vi "Build core.vi"(6 "Previous Build's Artifacts":refnum<class "Build Artifact.lvclass">[](array[class]), 7 "Progress":refnum<class "Progress.lvclass">, 8 "error in (no error)":errorcluster, 10 "Build Cache":refnum<class "Build Cache.lvclass">, 11 "Build Item in":refnum<class "Run Tests Step.lvclass">) -> (0 "error out":errorcluster, 1 "Explore Path":path, 2 "Build Results":T1, 4 "New Artifacts":refnum<class "Build Artifact.lvclass">[](array[class]))   [LabVIEW 2019, in "Caraya Library.lvlib" / "Run Tests Step.lvclass"]
doc: "Performs all the necessary build actions for the build step.\n\nCopyright: MGI 2016\nAuthor: Derek Trepanier"
uses:
  Run Tests Step.lvclass
  C:/Users/pasca/source/repos/mgi-solution-explorer-extensions/libs/Solution.lvlibp/Solution/Build Item/Build Step.lvclass
  libs/Solution.lvlibp/Solution/Progress/Progress.lvclass
  libs/Solution.lvlibp/Solution/Build Artifact/Build Artifact.lvclass
  libs/Solution.lvlibp/Solution/Build Item/Build Result.ctl
  libs/Solution.lvlibp/Solution/Build Cache/Build Cache.lvclass
  Run Tests Step.lvclass/Run Tests Step.ctl
  libs/Project.lvlibp/Project/Binary File/Binary File.lvclass
  C:/Users/pasca/source/repos/mgi-solution-explorer-extensions/libs/Solution.lvlibp/Solution/Build Artifact/Build Artifact.lvclass
  libs/Solution.lvlibp/Solution/Build Item/Build Step.lvclass
  <vilib>/addons/_JKI Toolkits/Caraya/Caraya.lvlib
  <vilib>/addons/_JKI Toolkits/Caraya/run-tests/Run Test (Scalar Path).vi
  Caraya Library.lvlib
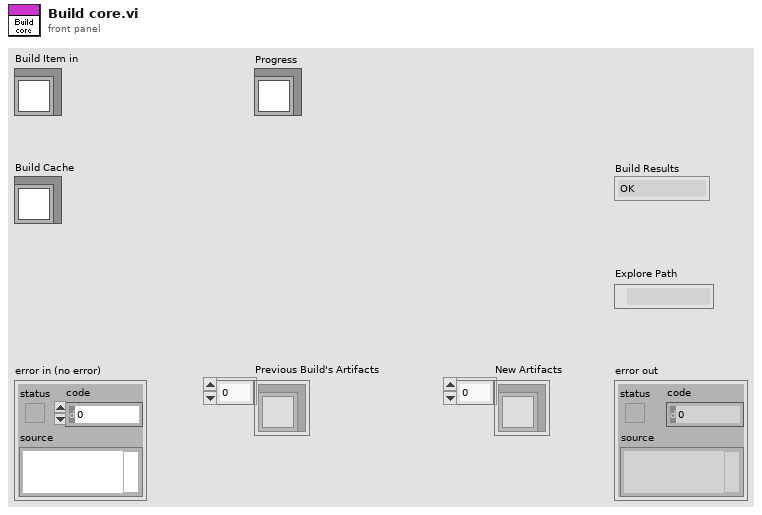
[diagram p1: front panel]
types:
  T1 = typedef "Solution.lvlibp/Build Step.lvclass/Build Result.ctl" = enum16{"OK", "Skipped", "Error"}
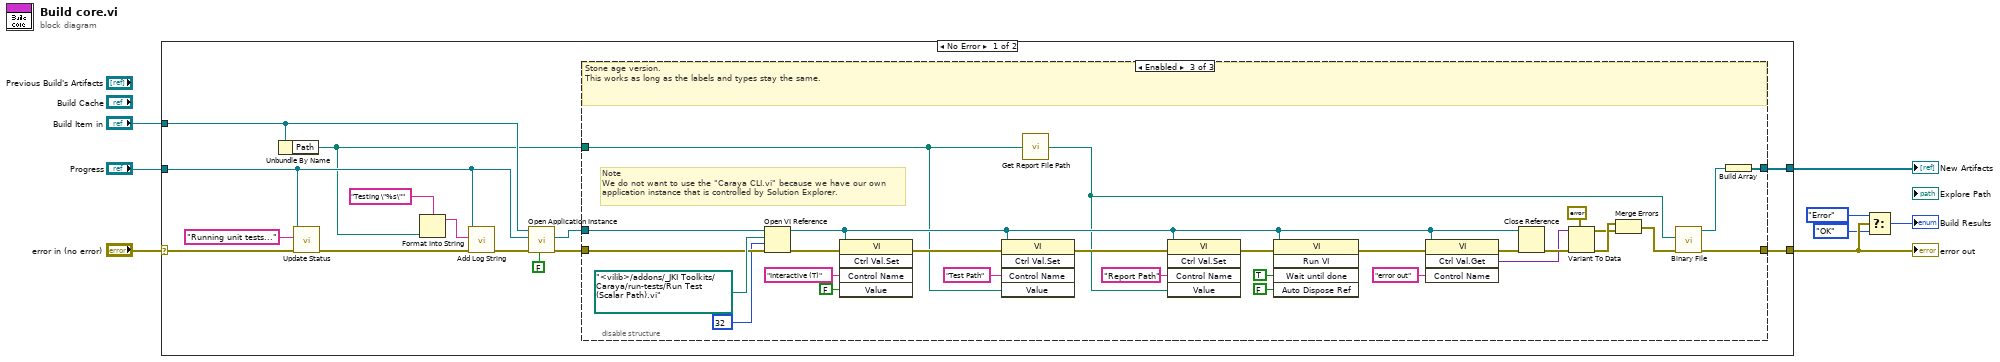
[diagram p0: block diagram]
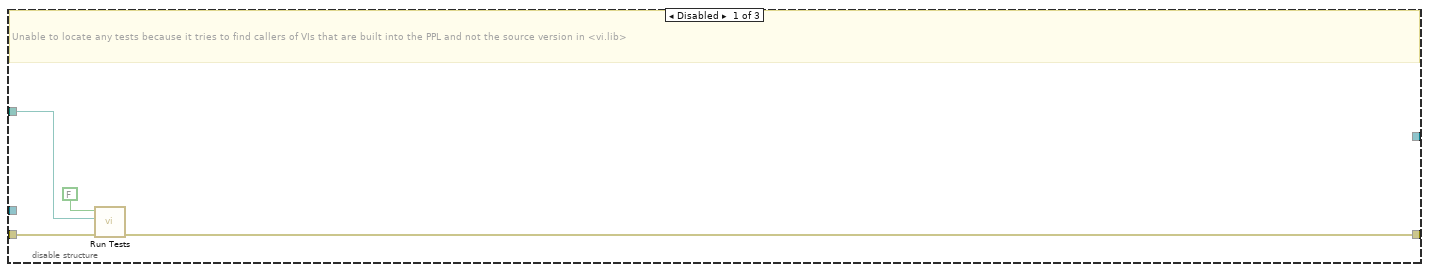
[diagram p2: hidden frame]
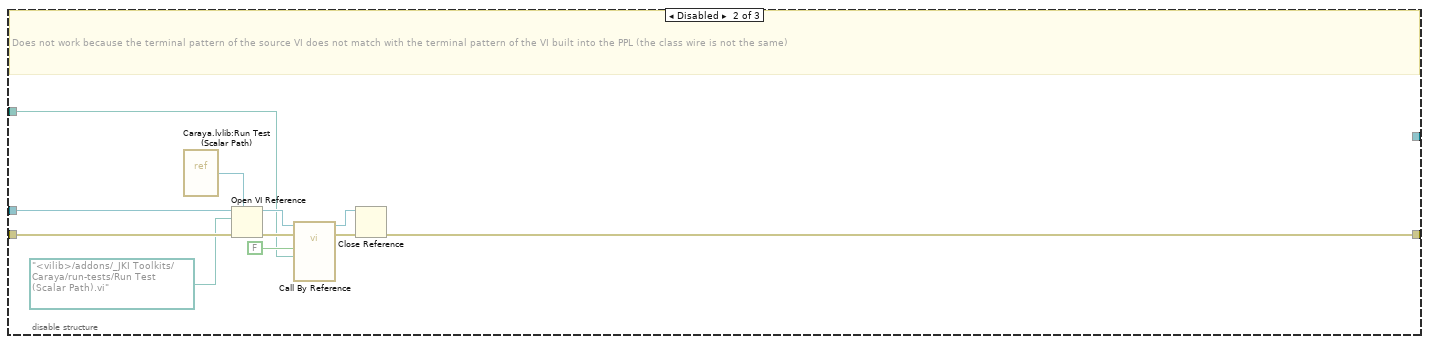
[diagram p3: hidden frame]
diagram:
  n1 = case shown="No Error" "error in (no error)" {
    selector: "error in (no error)" -> [w22 w67]
    tunnel: [w11 w67] -> w5
    tunnel: "Build Item in" -> [w16 _]
    tunnel: "Progress" -> [w15 _]
    tunnel: [w9 _] -> w1
    frame No Error {
      n2 = Unbundle By Name(w16) -> ("Path"=w12:path)
      n3 = call "Update Status.vi"("error in (no error)"=w22, "Status String"="Running unit tests...", "Progress in"=w15) -> ("error out"=w20:errorcluster)  [unwired: 8 in]
      n4 = Format Into String(format string="Testing \"%s\"" ("Log Item"), w12) -> (resulting string=w18:string)  [unwired: 2 in, 1 out]
      n5 = call "Add Log String.vi"("error in (no error)"=w20, "Log Item"=w18, "Progress in"=w15) -> ("error out"=w17:errorcluster)  [unwired: 8 in]
      n6 = call "Open Application Instance.vi"("64 Bit?"=FALSE, "error in (no error)"=w17, "Progress"=w15, "Build Step in"=w16) -> ("error out"=w13:errorcluster, "App ref"=w10:refnum<vi>)  [unwired: 6 in]
      n7 = disable-structure shown="Enabled" {
        disable-tunnel: w13 -> [w26 w37 w65]
        disable-tunnel: w12 -> [w24 w30 w39]
        disable-tunnel: [w23 w29 w51] -> w11
        disable-tunnel: w10 -> [_ w27 w55]
        disable-tunnel: [_ _ w49] -> w9
        frame Disabled {
          # "Unable to locate any tests because it tries to find callers of VIs that are built into the PPL and not the source version in <vi.lib>"
          n8 = call-poly <vilib>:"Run Tests.vi"("error in"=w26, "Test Path"=w24, "Interactive (T)"=FALSE) -> ("error out"=w23:errorcluster)  [unwired: 7 in, 1 out]
        }
        frame Disabled {
          # "Does not work because the terminal pattern of the source VI does not match with the terminal pattern of the VI built into the PPL (the class wire is not the same)"
          n9 = vi-ref "Caraya.lvlib:Run Test (Scalar Path).vi"() -> (w36:refnum<vi>)
          n10 = Open VI Reference(type specifier VI Refnum (for type only)=w36, application reference (local)=w27, vi path=path "<vilib>/addons/_JKI Toolkits/Caraya/run-tests/Run Test (Scalar Path).vi", error in (no error)=w37) -> (vi reference=w33:refnum<vi>, error out=w34:errorcluster)  [unwired: 2 in]
          n11 = call-by-ref "?"(reference=w33, error in=w34, "Test Path"=w30, "Interactive (T)"=FALSE) -> (reference out=w28:refnum<vi>, error out=w32:errorcluster)  [unwired: 8 in, 2 out]
          n12 = Close Reference(reference=w28, error in (no error)=w32) -> (error out=w29:errorcluster)
        }
        frame Enabled {
          # "Note\nWe do not want to use the \"Caraya CLI.vi\" because we have our own\napplication instance that is controlled by Solution Explorer."
          # "Stone age version.\nThis works as long as the labels and types stay the same."
          n13 = Open VI Reference(application reference (local)=w55, vi path=path "<vilib>/addons/_JKI Toolkits/Caraya/run-tests/Run Test (Scalar Path).vi", options=32, error in (no error)=w65) -> (vi reference=w47:refnum<vi>, error out=w61:errorcluster)  [unwired: 2 in]
          n14 = invoke class="VI" method="Ctrl Val.Set"(reference=w47, error in=w61, "Control Name"="Interactive (T)", "Value"=FALSE) -> (error out=w60:errorcluster)  [unwired: 1 in, 4 out]
          n15 = invoke class="VI" method="Ctrl Val.Set"(reference=w47, error in=w60, "Control Name"="Test Path", "Value"=w39) -> (error out=w57:errorcluster)  [unwired: 1 in, 4 out]
          n16 = call "Get Report File Path.vi"("Path"=w39) -> ("Report File"=w38:path)  [unwired: 1 in]
          n17 = invoke class="VI" method="Ctrl Val.Set"(reference=w47, error in=w57, "Control Name"="Report Path", "Value"=w38) -> (error out=w54:errorcluster)  [unwired: 1 in, 4 out]
          n18 = invoke class="VI" method="Run VI"(reference=w47, error in=w54, "Wait until done"=TRUE ("Wait Until Done"), "Auto Dispose Ref"=FALSE ("Auto Dispose Reference")) -> (error out=w64:errorcluster)  [unwired: 1 in, 4 out]
          n19 = invoke class="VI" method="Ctrl Val.Get"(reference=w47, error in=w64, "Control Name"="error out") -> (error out=w48:errorcluster, "Get Control Value Variant"=w43:variant)  [unwired: 1 in, 2 out]
          n20 = Close Reference(reference=w47, error in (no error)=w48) -> (error out=w52:errorcluster)
          n21 = Variant To Data(error in=w52, type=errorcluster {"status"=FALSE, "code"=0, "source"=""} ("error constant"), Variant=w43) -> (data=w41:errorcluster, error out=w44:errorcluster)
          n22 = Merge Errors(w44, w41) -> (w45:errorcluster)
          n23 = call "Binary File.vi"("error in (no error)"=w45, "File"=w38) -> ("error out"=w51:errorcluster, "Binary File out"=w50:refnum<class "Binary File.lvclass">)  [unwired: 8 in]
          n24 = Build Array(w50) -> (w49:refnum<class "Binary File.lvclass">[])
        }
      }
    }
    frame Error {
    }
  }
  "error out" <- w5
  "New Artifacts" <- w1
  n25 = Select(t=Build_Result."Error" ("Build Results"), s=w5, f=Build_Result."OK" ("Build Results")) -> (s? t:f=→"Build Results":T1)
